vi "9149_9220_AI_32.vi"() -> (3 "Array":fxp<+/-,24,5>[](array[numeric]))   [LabVIEW 2017]
uses:
  <vilib>/rvi/eio/common/nirviEmuTemplateMethod_errors.vi
  <vilib>/eio/EIONode/EIONode.xnode
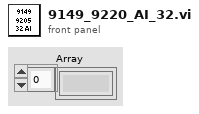
[diagram p1: front panel]
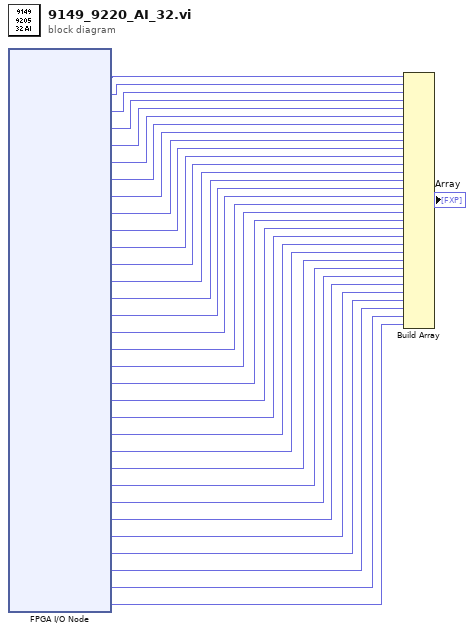
[diagram p0: block diagram]
diagram:
  n1 = xnode "FPGA I/O Node"() -> ("Mod3/AI0"=w1:fxp<+/-,24,5>, "Mod3/AI1"=w2:fxp<+/-,24,5>, "Mod3/AI2"=w3:fxp<+/-,24,5>, "Mod3/AI3"=w4:fxp<+/-,24,5>, "Mod3/AI4"=w5:fxp<+/-,24,5>, "Mod3/AI5"=w6:fxp<+/-,24,5>, "Mod3/AI6"=w7:fxp<+/-,24,5>, "Mod3/AI7"=w8:fxp<+/-,24,5>, "Mod3/AI8"=w9:fxp<+/-,24,5>, "Mod3/AI9"=w10:fxp<+/-,24,5>, "Mod3/AI10"=w11:fxp<+/-,24,5>, "Mod3/AI11"=w12:fxp<+/-,24,5>, "Mod3/AI12"=w13:fxp<+/-,24,5>, "Mod3/AI13"=w14:fxp<+/-,24,5>, "Mod3/AI14"=w15:fxp<+/-,24,5>, "Mod3/AI15"=w16:fxp<+/-,24,5>, "Mod4/AI0"=w17:fxp<+/-,24,5>, "Mod4/AI1"=w18:fxp<+/-,24,5>, "Mod4/AI2"=w19:fxp<+/-,24,5>, "Mod4/AI3"=w20:fxp<+/-,24,5>, "Mod4/AI4"=w21:fxp<+/-,24,5>, "Mod4/AI5"=w22:fxp<+/-,24,5>, "Mod4/AI6"=w23:fxp<+/-,24,5>, "Mod4/AI7"=w24:fxp<+/-,24,5>, "Mod4/AI8"=w25:fxp<+/-,24,5>, "Mod4/AI9"=w26:fxp<+/-,24,5>, "Mod4/AI10"=w27:fxp<+/-,24,5>, "Mod4/AI11"=w28:fxp<+/-,24,5>, "Mod4/AI12"=w29:fxp<+/-,24,5>, "Mod4/AI13"=w30:fxp<+/-,24,5>, "Mod4/AI14"=w31:fxp<+/-,24,5>, "Mod4/AI15"=w32:fxp<+/-,24,5>)  [unwired: 32 in, 32 out]
  n2 = Build Array(w1, w2, w3, w4, w5, w6, w7, w8, w9, w10, w11, w12, w13, w14, w15, w16, w17, w18, w19, w20, w21, w22, w23, w24, w25, w26, w27, w28, w29, w30, w31, w32) -> (→"Array":fxp<+/-,24,5>[])
